vi "Encode-Decode Checker.vi"() -> ()   [LabVIEW 2009]
panel:
  in  "Destination":T1={"Subsystem Id"=90.0, "Node Id"=1.0, "Component Id"=1.0}
  in  "Source":T1={"Subsystem Id"=3.0, "Node Id"=1.0, "Component Id"=1.0}
  out "Global OK":bool
  out "Individual OK":bool[](array[boolean])
  in  "Sequence Number (16 bits)":u16
  in  "Priority(40-41)":u8
  in  "Payload":string
  in  "Message Type (0-5)":u8
  in  "Header Compression (24-31)":u8
  in  "HC Length (32-39)":u8
  in  "HC flags (6-7)":u8
  in  "Data Size (8-23)":u16
  in  "Data Flags (46-47)":u8
  in  "Broadcast Flags (42-43)":u8
  in  "Ack/Nak (44-45)":u8
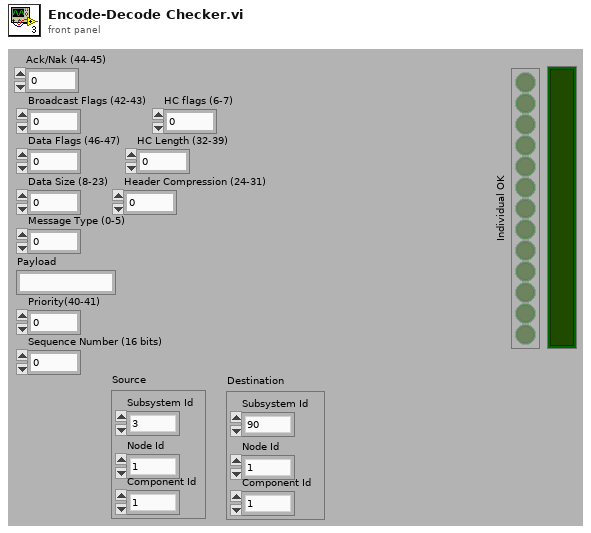
[diagram p1: front panel]
types:
  T1 = cluster{"Subsystem Id":dbl, "Node Id":dbl, "Component Id":dbl}
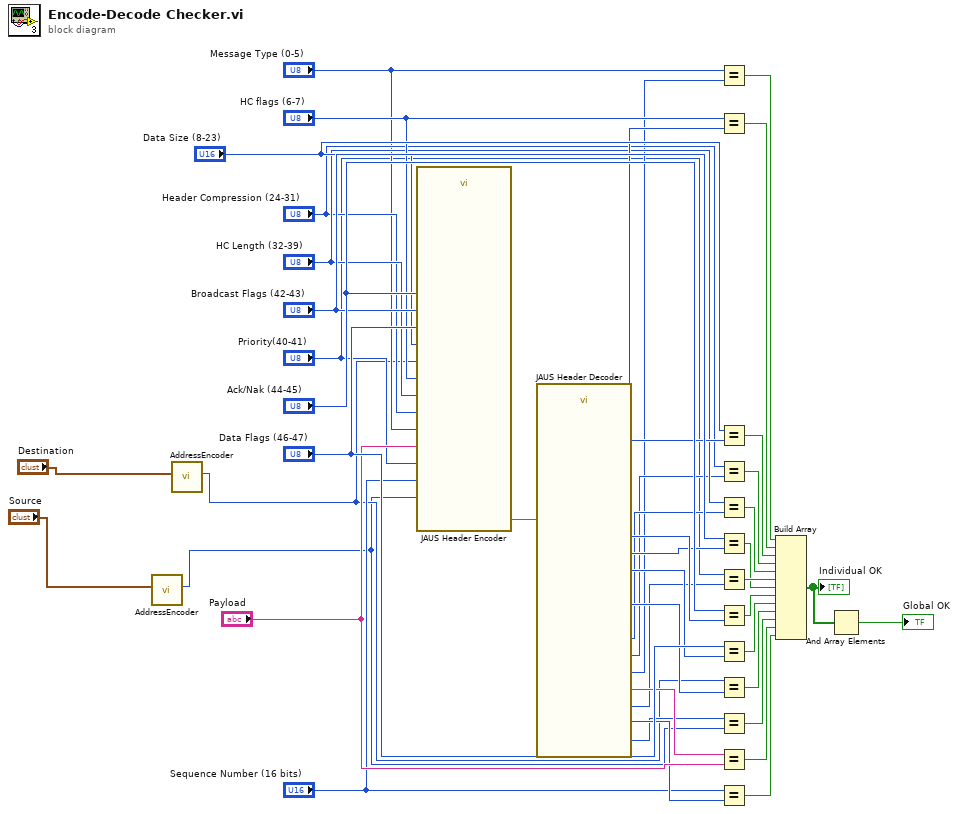
[diagram p0: block diagram]
diagram:
  n1 = call "AddressEncoder.vi"("Address Cluster"="Source") -> ("Address"=w1:u32)  [unwired: 10 in]
  n2 = call "AddressEncoder.vi"("Address Cluster"="Destination") -> ("Address"=w3:u32)  [unwired: 10 in]
  n3 = call "JAUS Header Encoder.vi"("Message Type (0-5)"="Message Type (0-5)", "HC flags (6-7)"="HC flags (6-7)", "Data Size (8-23)"="Data Size (8-23)", "HC Number (24-31)"="Header Compression (24-31)", "HC Length (32-39)"="HC Length (32-39)", "Priority(40-41)"="Priority(40-41)", "Sequence Number (16 bits)"="Sequence Number (16 bits)", "Broadcast Flags (42-43)"="Broadcast Flags (42-43)", "Payload"="Payload", "Source ID (80-95)"=w1, "Destination ID (48-79)"=w3, "Data Flags (46-47)"="Data Flags (46-47)", "Ack/Nak (44-45)"="Ack/Nak (44-45)") -> ("Encoded JAUS Message"=w44:string)  [unwired: 2 out]
  n4 = call "JAUS Header Decoder.vi"("Encoded JAUS Message"=w44) -> ("Message Type (0-5)"=w28:u8, "HC flags (6-7)"=w33:u8, "Data Size (8-23)"=w37:u16, "HC Number (24-31)"=w29:u8, "HC Length (32-39)"=w32:u8, "Priority(40-41)"=w23:u8, "Broadcast Flags (42-43)"=w40:u8, "Ack/Nak (44-45)"=w43:u8, "Data Flags (46-47)"=w38:u8, "Destination ID (48-79)"=w35:u32, "Source ID (80-95)"=w20:u32, "Payload"=w25:string, "Sequence Number (16 bits)"=w22:u16)  [unwired: 14 out]
  n5 = Equal?(x="Message Type (0-5)", y=w28) -> (x = y?=w17:bool)
  n6 = Equal?(x="HC flags (6-7)", y=w33) -> (x = y?=w16:bool)
  n7 = Equal?(x="Data Size (8-23)", y=w37) -> (x = y?=w15:bool)
  n8 = Equal?(x="Header Compression (24-31)", y=w29) -> (x = y?=w14:bool)
  n9 = Equal?(x="HC Length (32-39)", y=w32) -> (x = y?=w13:bool)
  n10 = Equal?(x="Broadcast Flags (42-43)", y=w40) -> (x = y?=w11:bool)
  n11 = Equal?(x="Priority(40-41)", y=w23) -> (x = y?=w12:bool)
  n12 = Equal?(x="Ack/Nak (44-45)", y=w43) -> (x = y?=w10:bool)
  n13 = Equal?(x="Data Flags (46-47)", y=w38) -> (x = y?=w9:bool)
  n14 = Equal?(x=w3, y=w35) -> (x = y?=w8:bool)
  n15 = Equal?(x=w20, y=w1) -> (x = y?=w7:bool)
  n16 = Equal?(x=w25, y="Payload") -> (x = y?=w6:bool)
  n17 = Equal?(x="Sequence Number (16 bits)", y=w22) -> (x = y?=w5:bool)
  n18 = Build Array(w17, w16, w15, w14, w13, w12, w11, w10, w9, w8, w7, w6, w5) -> (w19:bool[])
  "Individual OK" <- w19
  n19 = And Array Elements(Boolean array=w19) -> (logical AND=→"Global OK":bool)
